vi "Text _To_Speech.vi"() -> ()   [LabVIEW 2020]
uses:
  System.Speech
panel:
  in  "Path":path
  out "text to write":string
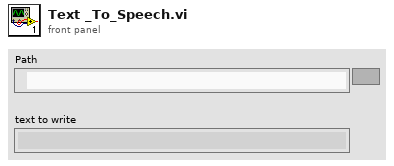
[diagram p1: front panel]
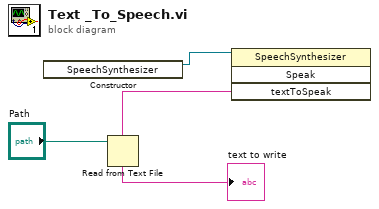
[diagram p0: block diagram]
diagram:
  n1 = constructor class="SpeechSynthesizer"() -> (reference out=w3:refnum<k24>)  [unwired: 3 in, 2 out]
  n2 = Read from Text File(file (use dialog)="Path") -> (text=w2:string)  [unwired: 3 in, 3 out]
  "text to write" <- w2
  n3 = invoke class="SpeechSynthesizer" method="Speak"(reference=w3, "textToSpeak"=w2) -> ()  [unwired: 2 in, 4 out]
